vi "AutonVision.vi"() -> (3 "Hot":bool)   [LabVIEW 2013]
uses:
  <vilib>/Rock Robotics/WPI/Camera/WPI_CameraImageSize.ctl
  Vision/TargetType.ctl
panel:
  in  "Score Limit":dbl=70.0
  in  "Image Size 2":T1=enum."320x240"
  in  "Color Components":T2={"Hue"={77.0, 75.0}, "Sat"={0.0, 255.0}, "Val"={237.0, 255.0}} {"Val" scale=0.0..255.0; "Sat" scale=0.0..255.0; "Hue" scale=0.0..255.0 scale format="%#_3g"}
  in  "Annotate":bool=TRUE
  in  "Enable Vision":bool=TRUE
  in  "error in (no error)":errorcluster
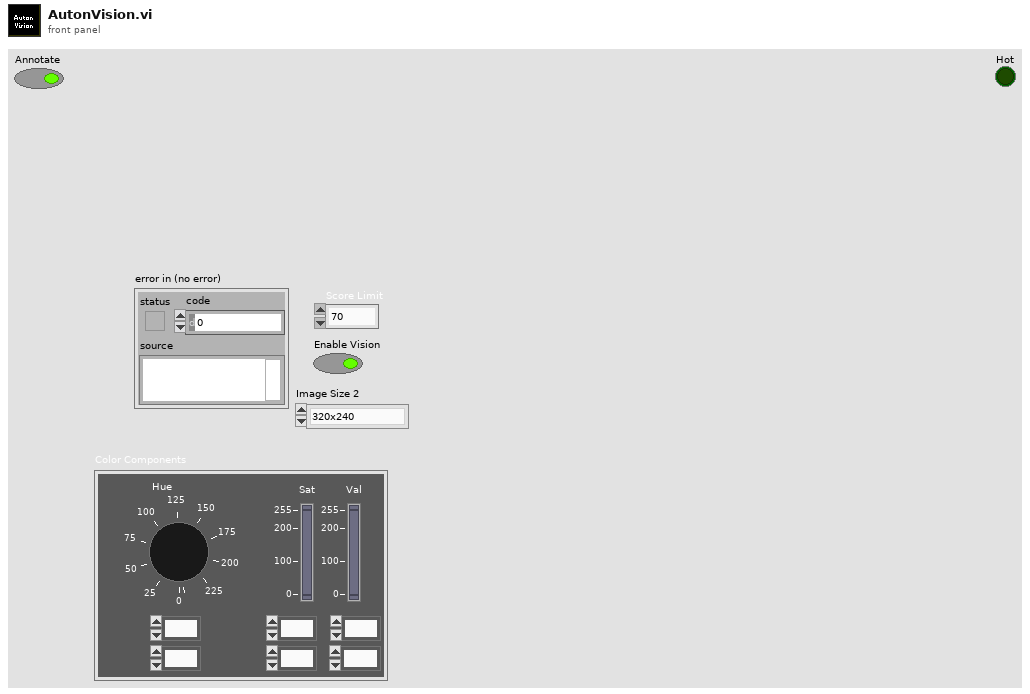
[diagram p1: front panel]
types:
  T1 = typedef "WPI_CameraImageSize.ctl" = enum16{"640x480", "320x240", "160x120"}
  T2 = cluster{"Hue":cluster{dbl, dbl}, "Sat":cluster{dbl, dbl}, "Val":cluster{dbl, dbl}}
  T3 = typedef "Image Type" = u32
  T4 = typedef "WPI_CameraDevRef.ctl" = cluster{"Camera Address":string, "CameraStatus":errorcluster, "Acquire Image Notifier":refnum<notifier>}
  T5 = typedef "IMAQ Image.ctl" = refnum<image>
  T6 = typedef "TargetType.ctl" = enum16{"Not Hot", "Hot"}
  T7 = cluster{"Horizontal":bool, "Aspect Score":dbl, "Rect Score":dbl, cluster{"Left":dbl, "Top":dbl, "Right":dbl, "Bottom":dbl}, "Equiv H":dbl, "Equiv V":dbl}[]
  T8 = cluster{"Scores":cluster{"Total":dbl, "Left":dbl, "Right":dbl, "Ratio":dbl, "Vertical":dbl, "index":i32, "State":T6}, "Verticals":cluster{"Horizontal?":bool, "Aspect Score":dbl, "Rect Score":dbl, cluster{"Left":dbl, "Top":dbl, "Right":dbl, "Bottom":dbl}, "Equiv H":dbl, "Equiv V":dbl}, "Horizontals":cluster{"Horizontal?":bool, "Aspect Score":dbl, "Rect Score":dbl, cluster{"Left":dbl, "Top":dbl, "Right":dbl, "Bottom":dbl}, "Equiv H":dbl, "Equiv V":dbl}, "Validated":bool}[]
  T9 = cluster{"Scores":cluster{"Total":dbl, "Left":dbl, "Right":dbl, "Ratio":dbl, "Vertical":dbl, "index":i32, "State":T6}, "Verticals":cluster{"Horizontal?":bool, "Aspect Score":dbl, "Rect Score":dbl, cluster{"Left":dbl, "Top":dbl, "Right":dbl, "Bottom":dbl}, "Equiv H":dbl, "Equiv V":dbl}, "Horizontals":cluster{"Horizontal?":bool, "Aspect Score":dbl, "Rect Score":dbl, cluster{"Left":dbl, "Top":dbl, "Right":dbl, "Bottom":dbl}, "Equiv H":dbl, "Equiv V":dbl}, "Validated":bool}
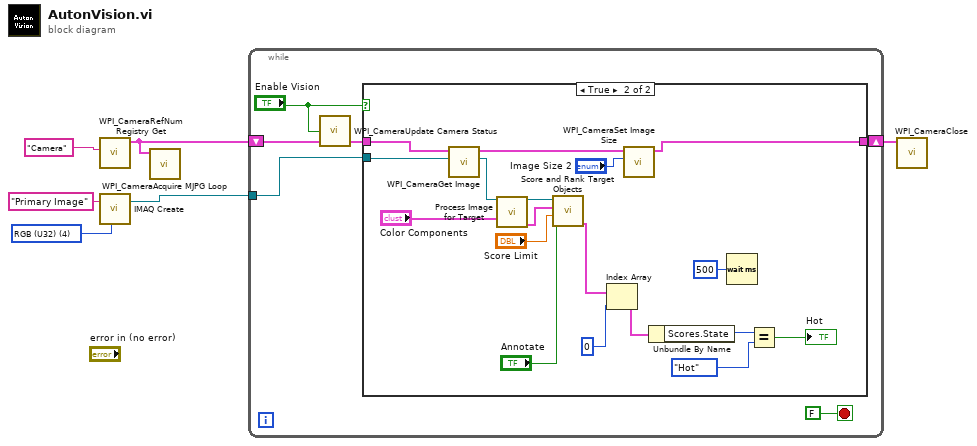
[diagram p0: block diagram]
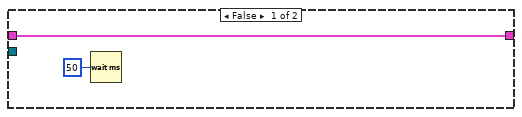
[diagram p2: hidden frame]
diagram:
  w6 = T3 4 items=["Grayscale (U8)", "Grayscale (I16)", "Grayscale (SGL)", "Complex (CSG)", "RGB (U32)", "HSL (U32)", "RGB (U64)"] ("Image Type")
  n1 = call <vilib>:"WPI_CameraRefNum Registry Get.vi"("refnum name"="Camera") -> ("CameraDevRef"=w2:T4)  [unwired: 9 in, 1 out]
  n2 = call "IMAQ Create"("Image Name"="Primary Image", "Image Type"=w6) -> ("New Image"=w4:T5)  [unwired: 2 in, 2 out]
  n3 = call <vilib>:"WPI_CameraAcquire MJPG Loop.vi"("CameraDevRef"=w2) -> ()  [unwired: 11 in]
  n4 = while {
    tunnel: w4 -> [w12]
    shift-right: [w11] -> w3
    shift-left: w2 -> [w10]
    stop <- FALSE stop-if-true
    n5 = call <vilib>:"WPI_CameraUpdate Camera Status.vi"("CameraDevRef In"=w10, "Enable Vision"="Enable Vision") -> ("CameraDevRef Out"=w9:T4)  [unwired: 3 in]
    n6 = case shown="True" "Enable Vision" {
      tunnel: w12 -> [_ w31]
      tunnel: [w14 w32] -> w11
      tunnel: w9 -> [w14 w30]
      frame False {
        n7 = Wait (ms)(milliseconds to wait=u32 50) -> ()  [unwired: 1 out]
      }
      frame True {
        n8 = call <vilib>:"WPI_CameraGet Image.vi"("Image"=w31, "CameraDevRef"=w30) -> ("Image Out"=w28:T5, "CameraDevRef Out"=w29:T4)  [unwired: 1 in, 7 out]
        n9 = call "Process Image for Target.vi"("Src Image"=w28, "Color Components"="Color Components") -> ("Src Image Out"=w27:T5, "Particles"=w26:T7)  [unwired: 11 in, 1 out]
        n10 = call "Score and Rank Target Objects.vi"("Annotate"="Annotate", "Score Limit"="Score Limit", "Particles"=w26, "Image in"=w27) -> ("Target Info"=w21:T8)  [unwired: 6 in, 1 out]
        n11 = Index Array(array=w21, index=0) -> (element=w19:T9)
        n12 = call <vilib>:"WPI_CameraSet Image Size.vi"("Image Size"="Image Size 2", "CameraDevRef"=w29) -> ("CameraDevRef Out"=w32:T4)  [unwired: 1 in, 8 out]
        n13 = Unbundle By Name(w19) -> ("Scores.State"=w18:T6)
        n14 = Wait (ms)(milliseconds to wait=u32 500) -> ()  [unwired: 1 out]
        n15 = Equal?(x=w18, y=TargetType."Hot" ("Scores.State")) -> (x = y?=→"Hot":bool)
      }
    }
  }
  n16 = call <vilib>:"WPI_CameraClose.vi"("CameraDevRef"=w3) -> ()  [unwired: 1 in, 10 out]
